vi "get_numeric_type_info.vi"(8 "error in (no error)":errorcluster, 10 "Refnum":refnum<vi>) -> (0 "error out":errorcluster, 1 "Precision":string, 2 "max":string, 3 "Min":string)   [LabVIEW 2015]
panel:
  in  "DummyNumeric 2":refnum<vi>
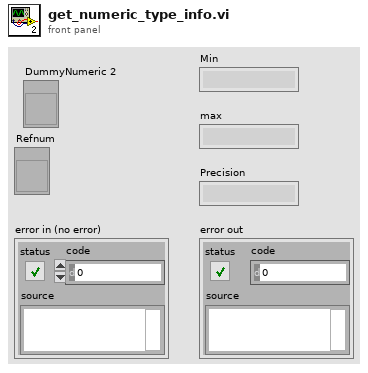
[diagram p1: front panel]
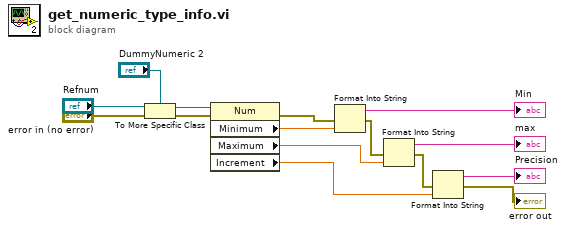
[diagram p0: block diagram]
diagram:
  n1 = To More Specific Class(target class="DummyNumeric 2", reference="Refnum", error in="error in (no error)") -> (specific class reference=w15:refnum<vi>, error out=w12:errorcluster)
  n2 = property class="Num"(reference=w15, error in=w12) -> (error out=w4:errorcluster, "Minimum"=w7:dbl, "Maximum"=w6:dbl, "Increment"=w5:dbl)  [unwired: 1 out]
  n3 = Format Into String(error in=w4, w7) -> (resulting string=→"Min":string, error out=w3:errorcluster)  [unwired: 2 in]
  n4 = Format Into String(error in=w3, w6) -> (resulting string=→"max":string, error out=w2:errorcluster)  [unwired: 2 in]
  n5 = Format Into String(error in=w2, w5) -> (resulting string=→"Precision":string, error out=→"error out":errorcluster)  [unwired: 2 in]
